vi "while_l0.vi"() -> ()   [LabVIEW 2010]
panel:
  out "Boolean":bool
  in  "stop":bool
  in  "Delay (ms)":dbl(slide)=25.71428571428571 scale=0.0..25.0
  out "Waveform Chart":dbl(graph)
  in  "Width":dbl(knob)=20.0 scale=0.0..20.0
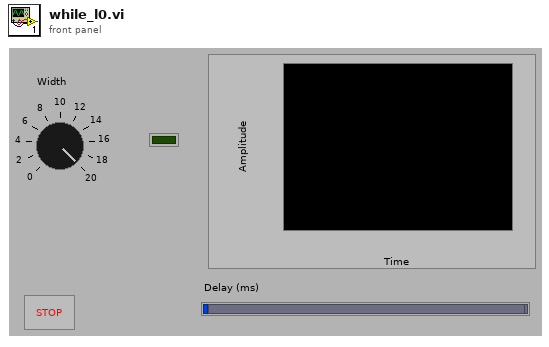
[diagram p1: front panel]
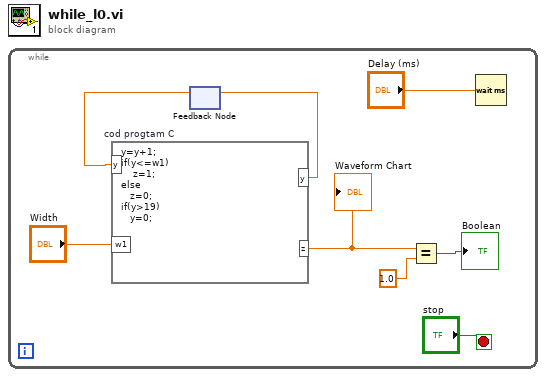
[diagram p0: block diagram]
diagram:
  n1 = while {
    stop <- "stop" stop-if-true
    n2 = feedback #1() -> (w1:dbl)  [unwired: 1 in]
    n3 = formula code="y=y+1;\nif(y<=w1)\n    z=1;\nelse\n   z=0;\nif(y>19)\n   y=0;" "cod progtam C"("w1"="Width", "y"=w1) -> ("z"=w4:dbl, "y"=w2:dbl)
    "Waveform Chart" <- w4
    n4 = feedback-in #1(w2) -> ()
    n5 = Equal?(x=w4, y=1.0) -> (x = y?=→"Boolean":bool)
    n6 = Wait (ms)(milliseconds to wait="Delay (ms)") -> ()  [unwired: 1 out]
  }
